vi "PortDictionary.vi"(9 "Tasks":enum16{"Read", "Write"}(ring), 11 "Ports in":T1(array[cluster])) -> (3 "Ports out":T1(array[cluster]))   [LabVIEW 2019]
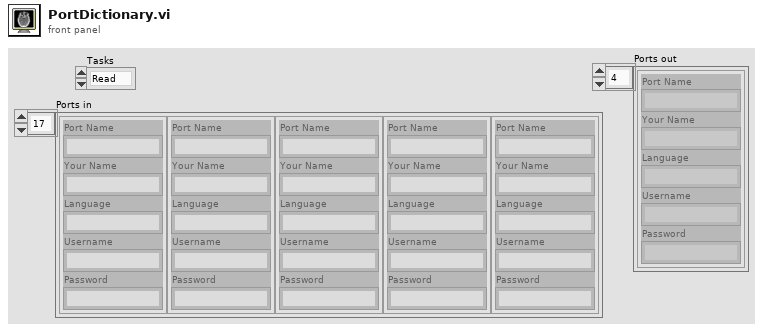
[diagram p1: front panel]
types:
  T1 = cluster{"Port Name":string, "Your Name":string, "Language":string, "Username":string, "Password":string}[]
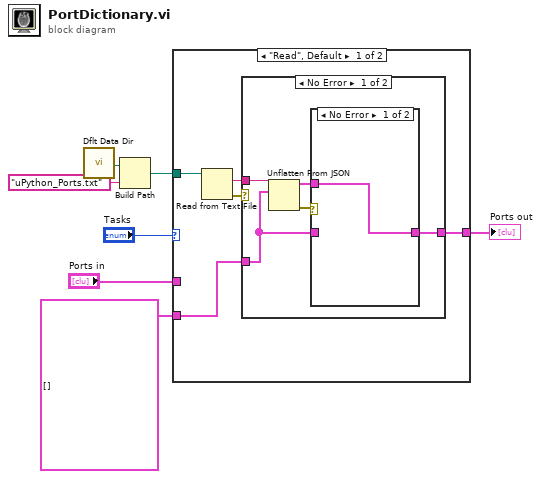
[diagram p0: block diagram]
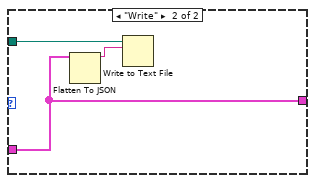
[diagram p4: hidden frame]
diagram:
  n1 = call <vilib>:"Dflt Data Dir.vi"() -> ("App:Default Data Directory"=w7:path)
  n2 = Build Path(base path=w7, name or relative path="uPython_Ports.txt") -> (appended path=w4:path)
  n3 = case shown="\"Read\", Default" "Tasks" {
    tunnel: w4 -> [w12 w23]
    tunnel: [w10 w21] -> w3
    tunnel: T1 [] -> [w9 _]
    tunnel: "Ports in" -> [_ w21]
    frame "Read", Default {
      n4 = Read from Text File(file (use dialog)=w12) -> (text=w8:string, error out=w11:errorcluster)  [unwired: 3 in, 2 out]
      n5 = case shown="No Error" w11 {
        tunnel: [w15 w20] -> w10
        tunnel: w9 -> [w13 w20]
        tunnel: w8 -> [w17 _]
        frame No Error {
          n6 = Unflatten From JSON(JSON string=w17, type and defaults=w13) -> (value=w14:T1, error out=w16:errorcluster)  [unwired: 5 in]
          n7 = case shown="No Error" w16 {
            tunnel: [w18 w19] -> w15
            tunnel: w14 -> [w18 _]
            tunnel: w13 -> [_ w19]
            frame No Error {
            }
            frame Error {
            }
          }
        }
        frame Error {
        }
      }
    }
    frame "Write" {
      n8 = Flatten To JSON(anything=w21) -> (JSON string=w22:string)  [unwired: 2 in, 1 out]
      n9 = Write to Text File(file (use dialog)=w23, text=w22) -> ()  [unwired: 2 in, 3 out]
    }
  }
  "Ports out" <- w3
